vi "Read Inputs from system.vi"(8 "error in":errorcluster, 11 "RTResourceUtilitzation runtime in":refnum<class "RTResourceUtilitzation runtime.lvclass">) -> (0 "error out":errorcluster, 2 "Inputs from system":T1, 3 "RTResourceUtilitzation runtime out":refnum<class "RTResourceUtilitzation runtime.lvclass">)   [LabVIEW 2014, in "RTResourceUtilitzation runtime.lvclass"]
uses:
  RTResourceUtilitzation runtime.lvclass
  configuration/input data indices.ctl
  RTResourceUtilitzation runtime.lvclass/RTResourceUtilitzation runtime.ctl
  configuration/RTResourceUtilitzation configuration.lvclass
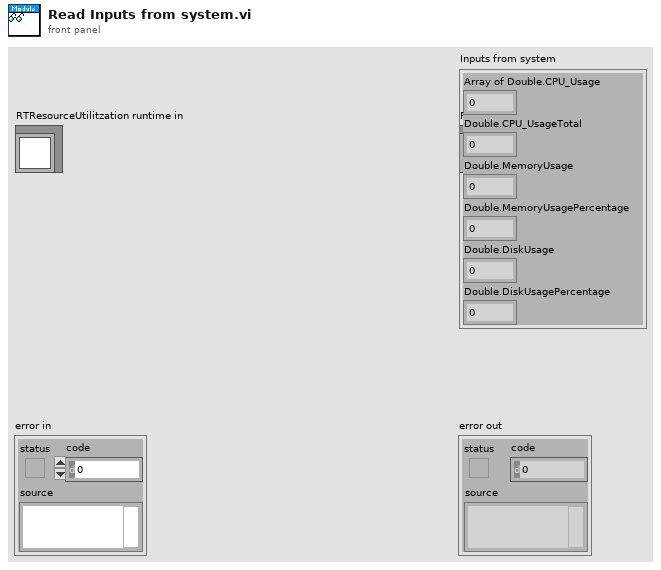
[diagram p1: front panel]
types:
  T1 = typedef "RTResourceUtilitzation configuration.lvclass/input data indices.ctl" = cluster{"Array of Double.CPU_Usage":i32, "Double.CPU_UsageTotal":i32, "Double.MemoryUsage":i32, "Double.MemoryUsagePercentage":i32, "Double.DiskUsage":i32, "Double.DiskUsagePercentage":i32}
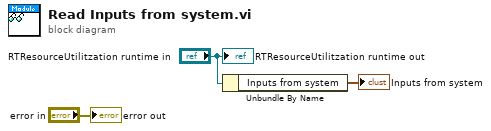
[diagram p0: block diagram]
diagram:
  n1 = Unbundle By Name("RTResourceUtilitzation runtime in") -> ("Inputs from system"=→"Inputs from system":T1)
  "error out" <- "error in"
  "RTResourceUtilitzation runtime out" <- "RTResourceUtilitzation runtime in"
